vi "COMI SD502 Set Counter.vi"(7 "nClkSource":u32, 9 "nMode":i32, 10 "ch":i32, 11 "hDevice":u32) -> (3 "hDevice out":u32)   [LabVIEW 2017, in "Comidll.lvlib"]
doc: "void (COMI_SD502_SetCounter) (HANDLE hDevice, int ch, int nMode, unsigned int nClkSource);"
uses:
  <userlib>/Comidll/Comidll.lvlib
  <userlib>/Comidll/Comidll.dll
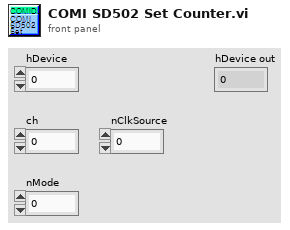
[diagram p1: front panel]
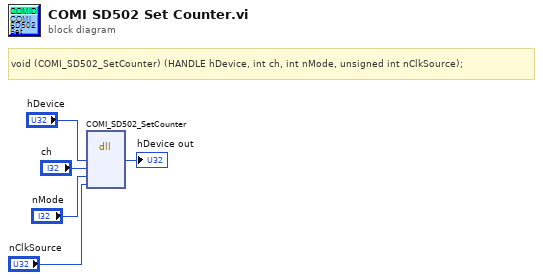
[diagram p0: block diagram]
diagram:
  # "void\t(COMI_SD502_SetCounter) (HANDLE hDevice, int ch, int nMode, unsigned int nClkSource);"
  n1 = dll-call lib="C:/Program Files/National Instruments/LabVIEW 2017/user.lib/Comidll/Comidll.*" fn="COMI_SD502_SetCounter"("hDevice"="hDevice", "ch"="ch", "nMode"="nMode", "nClkSource"="nClkSource") -> ("hDevice"=→"hDevice out":u32)  [unwired: 7 in, 2 out]
